vi "Picture size arrays.vi"(11 "Draw Area Size":T1) -> (2 "Center":dbl[](array[numeric]), 3 "Size":dbl[](array[numeric]))   [LabVIEW 2023]
doc: "Compute the size and center of the picture control"
uses:
  <vilib>/Utility/miscctls.llb/LVBoundsTypeDef.ctl
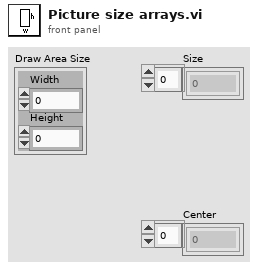
[diagram p1: front panel]
types:
  T1 = typedef "LVBoundsTypeDef.ctl" = cluster{"Width":u32, "Height":u32}
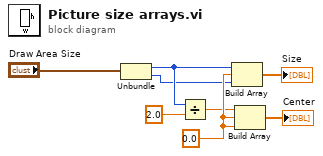
[diagram p0: block diagram]
diagram:
  w6 = 0.0
  n1 = Unbundle("Draw Area Size") -> ("Width"=w5:u32, "Height"=w1:u32)
  n2 = Divide(x=w5, y=2.0) -> (x/y=w4:dbl)
  n3 = Build Array(w5, w6, w1) -> (→"Size":dbl[])
  n4 = Build Array(w4, w6, w6) -> (→"Center":dbl[])
